vi "TOOLweb MESSWERTE.vi"(8 "error in (no error)":errorcluster caption="Fehler (Eingang, kein Fehler)", 9 "IP-Adresse (localhost)":string="127.0.0.1", 11 "Anzahl Gase":i32=18) -> (0 "Status":sgl[](array[numeric]), 1 "Diagnose":T2, 2 "gas#label":string[](array[string]), 5 "Zeitstempel":timestamp, 7 "Einstellungen":T1)   [LabVIEW 2020, in "FT-IR.lvlib" / "TOOLweb Interface.lvlib"]
doc: "Holt mit einer HTTP-POST-Anforderung gemäß TOOLweb-Protokoll die Gasmesswerte als Signalverläufe mit Gasnamen als Attribut \"NI_ChannelName\" und Zeitstempel vom MKS MultiGas 2030 Analyzer. Zwei Arrays mit den Gasnamen (Strings) und Gaskonzentrationsfehlern (DBL) werden zusätzlich bereitgestellt.\n\nAlle Daten werden zeitsparend in einem einzigen Poll Request zusammengefasst, damit nur einmal eine TCP/IP-Verbindung geöffnet werden muss.\n\nDer Ergebnis-Datentyp\"TOOLweb Signalverläufe\" ist als Typdefinitionen in der Bibliothek \"Datentypen\" enthalten\".\n\nFalls \"Anzahl Gase\" unverbunden bleibt, wird der Standardwert 18 verwendet.\n \nFalls der TOOLWeb-Server nicht auf demselben Rechner arbeitet, kann mit \"IP-Adresse\" eine beliebiger Host adressiert werden. Ein unverbundener Eingang spricht den lokalen Host an."
uses:
  TOOLweb Interface.lvlib
  TOOLweb Diagnose.ctl
  TOOLweb Einstellungen.ctl
  Stoerungen/Stoerungen Messgeraet/Aktionen Kommunikation Stoerung.ctl
  Get Spectra/Aktion FGV Background-Daten.ctl
  Aktion FGV Rezepte wechseln.ctl
  Span/Aktion FGV Span.ctl
  Aktionen EVID-Codes.ctl
  TOOLweb Interface Hilfs-VIs.lvlib
  Typdefinitionen.lvlib
  Stoerungen/Stoerungen.lvlib
  Get Spectra/Get Spectra.lvlib
  FT-IR.lvlib
  Span/Spanfaktor.lvlib
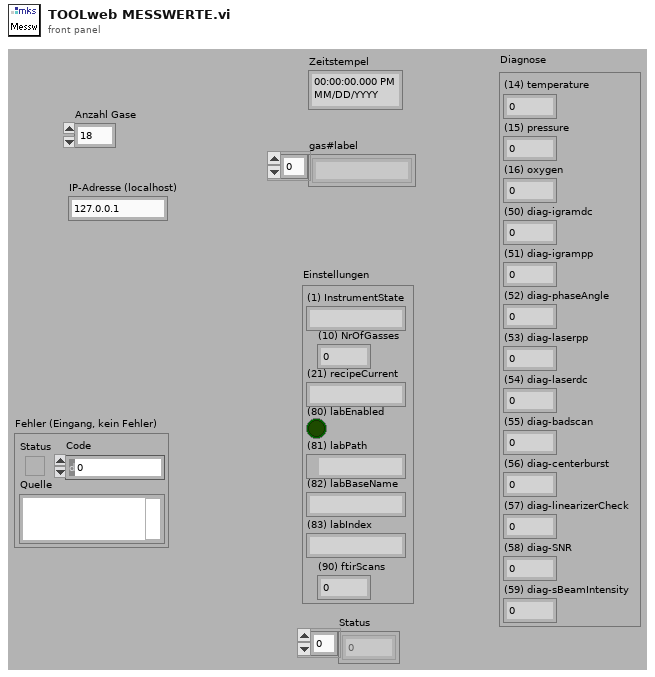
[diagram p1: front panel]
types:
  T1 = typedef "FT-IR.lvlib/TOOLweb Interface.lvlib/Typdefinitionen.lvlib/TOOLweb Einstellungen.ctl" = cluster{"(1) InstrumentState":string, "(10) NrOfGasses":i32, "(21) recipeCurrent":string, "(80) labEnabled":bool, "(81) labPath":path, "(82) labBaseName":string, "(83) labIndex":string, "(90) ftirScans":i32}
  T2 = typedef "FT-IR.lvlib/TOOLweb Interface.lvlib/Typdefinitionen.lvlib/TOOLweb Diagnose.ctl" = cluster{"(14) temperature":sgl, "(15) pressure":sgl, "(16) oxygen":sgl, "(50) diag-igramdc":sgl, "(51) diag-igrampp":sgl, "(52) diag-phaseAngle":sgl, "(53) diag-laserpp":sgl, "(54) diag-laserdc":sgl, "(55) diag-badscan":sgl, "(56) diag-centerburst":sgl, "(57) diag-linearizerCheck":sgl, "(58) diag-SNR":sgl, "(59) diag-sBeamIntensity":sgl}
  T3 = typedef "FT-IR.lvlib/Aktionen EVID-Codes.ctl" = enum16{"lesen", "setzen", "laden", "speichern", "1Hz/5Hz", "Smoothing", "Rolling Average"}
  T4 = typedef "FT-IR.lvlib/Spanfaktor.lvlib/Aktion FGV Span.ctl" = enum16{"lesen", "Span", "Seite aktiv", "Offset", "FGV aktualisiert", "Aktualisierung aufheben"}
  T5 = typedef "FT-IR.lvlib/Aktion FGV Rezepte wechseln.ctl" = enum16{"lesen", "Rezepte", "Rezeptindex", "Diesel", "Gasoline", "NCG", "laden", "speichern", "AK/Man"}
  T6 = typedef "FT-IR.lvlib/Get Spectra.lvlib/Aktion FGV Background-Daten.ctl" = enum16{"lesen", "schreiben", "Background aktiv", "Referenz", "laden", "speichern", "Plot sichtbar"}
  T7 = typedef "Stoerungen.lvlib/Aktionen Kommunikation Stoerung.ctl" = enum16{"lesen", "init", "FT-IR Komm", "FT-IR Betriebsart", "FT-IR Hintergrund", "cRIO Komm", "PNS Komm", "Dichtheitstest", "Life Bit", "FTIR Komm AK", "PMA Komm", "FID Komm", "PMA Cal", "FID Ch4 Cal", "FID THC Cal", "Cal Timeout", "VFS 1 Komm", "VFS 2 Komm", "VFS 3 Komm", "VFS 4 Komm", "TRE 08 Komm", "CG-Test vorzeitig", "CG-Test Span 1", "CG-Test Span 2", "CG-Test Span 3", "CG-Test Messgas", "CG-Test löschen", "Test", "Amium AK", "AK Recept konfig", "AK Name konfig", "AK EKFG konfig"}
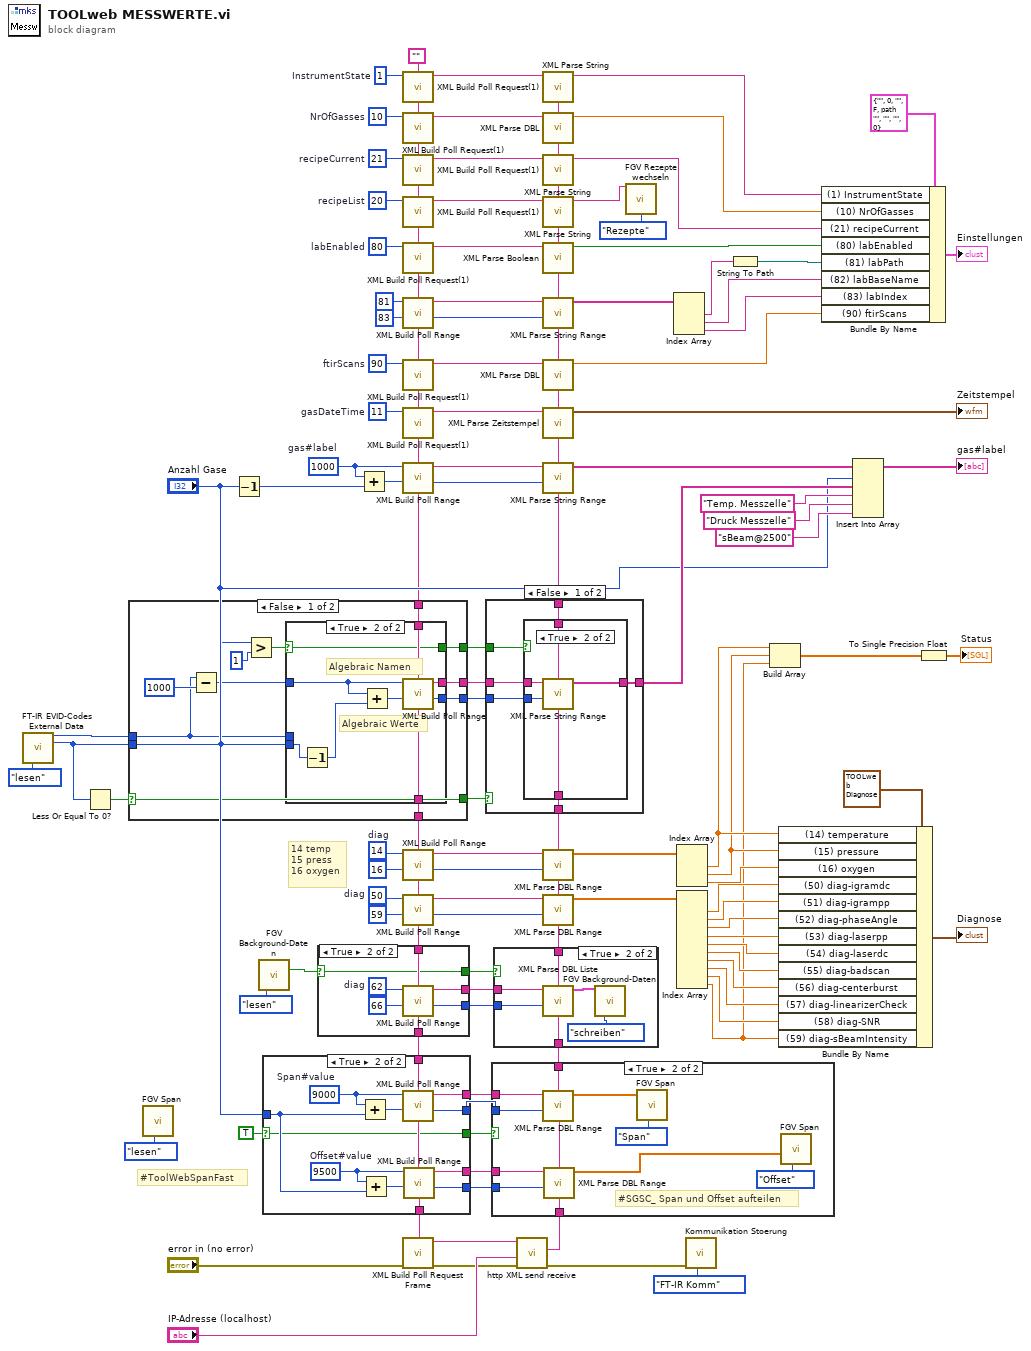
[diagram p0: block diagram]
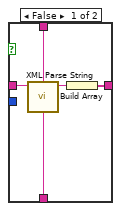
[diagram p2: hidden frame]
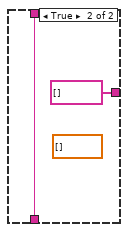
[diagram p3: hidden frame]
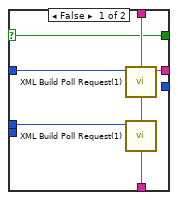
[diagram p4: hidden frame]
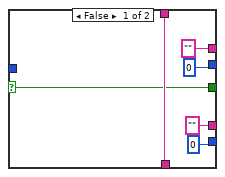
[diagram p7: hidden frame]
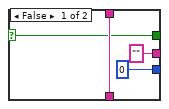
[diagram p9: hidden frame]
diagram:
  w29 = 20  # recipeList
  w54 = 14  # diag
  w81 = 90  # ftirScans
  w86 = 1  # InstrumentState
  w88 = 80  # labEnabled
  w89 = 21  # recipeCurrent
  w90 = 10  # NrOfGasses
  w103 = 50  # diag
  w126 = 1000  # gas#label
  w127 = 11  # gasDateTime
  # "#ToolWebSpanFast"
  # "14 temp\n15 press\n16 oxygen"
  n1 = call "FT-IR EVID-Codes External Data.vi"("Aktionen"=Aktionen_EVID-Codes."lesen") -> ("Startadresse"=w7:i32, "Anzahl"=w6:i32)  [unwired: 9 in, 4 out]
  n2 = Less Or Equal To 0?(x=w6) -> (x <= 0?=w5:bool)
  n3 = call "FGV Span.vi"("Aktion"=Aktion_FGV_Span."lesen") -> ()  [unwired: 7 in, 4 out]
  n4 = Decrement(x="Anzahl Gase") -> (x-1=w120:i32)
  n5 = call "FGV Background-Daten.vi"("Aktion"=Aktion_FGV_Background-Daten."lesen") -> ("Background aktiv"=w37:bool)  [unwired: 7 in, 7 out]
  n6 = Add(x=w126, y=w120) -> (x+y=w124:i32)
  n7 = call "XML Build Poll Request(1).vi"("XML-Message alt"="", "EVID-Nummer"=w86) -> ("Attribut Name"=w85:string, "XML-Message neu"=w78:string)  [unwired: 6 out]
  n8 = call "XML Build Poll Request(1).vi"("XML-Message alt"=w78, "EVID-Nummer"=w90) -> ("Attribut Name"=w91:string, "XML-Message neu"=w74:string)  [unwired: 6 out]
  n9 = call "XML Build Poll Request(1).vi"("XML-Message alt"=w74, "EVID-Nummer"=w89) -> ("Attribut Name"=w87:string, "XML-Message neu"=w28:string)  [unwired: 6 out]
  n10 = call "XML Build Poll Request(1).vi"("XML-Message alt"=w28, "EVID-Nummer"=w29) -> ("Attribut Name"=w30:string, "XML-Message neu"=w27:string)  [unwired: 6 out]
  n11 = call "XML Build Poll Request(1).vi"("XML-Message alt"=w27, "EVID-Nummer"=w88) -> ("Attribut Name"=w82:string, "XML-Message neu"=w61:string)  [unwired: 6 out]
  n12 = call "XML Build Poll Range.vi"("XML-Message alt"=w61, "von EVID-Nr"=81, "bis EVID-Nr"=83) -> ("Attribut Name (Range)"=w66:string, "Anzahl Elemente"=w67:i32, "XML-Message neu"=w59:string)  [unwired: 1 in, 3 out]
  n13 = call "XML Build Poll Request(1).vi"("XML-Message alt"=w59, "EVID-Nummer"=w81) -> ("Attribut Name"=w80:string, "XML-Message neu"=w70:string)  [unwired: 6 out]
  n14 = call "XML Build Poll Request(1).vi"("XML-Message alt"=w70, "EVID-Nummer"=w127) -> ("Attribut Name"=w125:string, "XML-Message neu"=w93:string)  [unwired: 6 out]
  n15 = call "XML Build Poll Range.vi"("XML-Message alt"=w93, "von EVID-Nr"=w126, "bis EVID-Nr"=w124) -> ("Attribut Name (Range)"=w123:string, "Anzahl Elemente"=w122:i32, "XML-Message neu"=w3:string)  [unwired: 1 in, 3 out]
  n16 = case shown="False" w5 {
    selector: w5 -> [w128 w157]
    tunnel: [w139 _] -> w10
    tunnel: [w138 _] -> w9
    tunnel: w3 -> [w137 w156]
    tunnel: [w136 w156] -> w45
    tunnel: [w133 _] -> w8
    tunnel: w7 -> [w131 _]
    tunnel: w6 -> [w129 _]
    tunnel: [w128 w157] -> w4
    frame False {
      n17 = Subtract(x=w131, y=1000) -> (x-y=w130:i32)
      n18 = Greater?(x=w129, y=1) -> (0:w135:bool)
      n19 = case shown="True" w135 {
        selector: w135 -> [w140 w151]
        tunnel: w131 -> [w146 _]
        tunnel: w129 -> [_ w149]
        tunnel: [w144 w155] -> w139
        tunnel: [_ w154] -> w138
        tunnel: w137 -> [w143 w152]
        tunnel: [w141 w147] -> w136
        tunnel: [w140 w151] -> w133
        tunnel: w130 -> [w145 w150]
        frame False {
          n20 = call "XML Build Poll Request(1).vi"("XML-Message alt"=w143, "EVID-Nummer"=w145) -> ("Attribut Name"=w144:string, "XML-Message neu"=w142:string)  [unwired: 6 out]
          n21 = call "XML Build Poll Request(1).vi"("XML-Message alt"=w142, "EVID-Nummer"=w146) -> ("XML-Message neu"=w141:string)  [unwired: 7 out]
        }
        frame True {
          # "Algebraic Werte"
          # "Algebraic Namen"
          n22 = Decrement(x=w149) -> (x-1=w148:i32)
          n23 = Add(x=w150, y=w148) -> (x+y=w153:i32)
          n24 = call "XML Build Poll Range.vi"("XML-Message alt"=w152, "von EVID-Nr"=w150, "bis EVID-Nr"=w153) -> ("Attribut Name (Range)"=w155:string, "Anzahl Elemente"=w154:i32, "XML-Message neu"=w147:string)  [unwired: 1 in, 3 out]
        }
      }
    }
    frame True {
    }
  }
  n25 = call "XML Build Poll Range.vi"("XML-Message alt"=w45, "von EVID-Nr"=w54, "bis EVID-Nr"=16) -> ("Attribut Name (Range)"=w52:string, "Anzahl Elemente"=w51:i32, "XML-Message neu"=w50:string)  [unwired: 1 in, 3 out]
  n26 = call "XML Build Poll Range.vi"("XML-Message alt"=w50, "von EVID-Nr"=w103, "bis EVID-Nr"=59) -> ("Attribut Name (Range)"=w105:string, "Anzahl Elemente"=w106:i32, "XML-Message neu"=w44:string)  [unwired: 1 in, 3 out]
  n27 = case shown="True" w37 {
    selector: w37 -> [w158 w162]
    tunnel: w44 -> [w161 w168]
    tunnel: [w161 w167] -> w22
    tunnel: ["" ("Attribut Name (Range)") w164] -> w39
    tunnel: [0 ("Anzahl Elemente") w163] -> w38
    tunnel: [w158 w162] -> w36
    frame False {
    }
    frame True {
      w166 = 62  # diag
      n28 = call "XML Build Poll Range.vi"("XML-Message alt"=w168, "von EVID-Nr"=w166, "bis EVID-Nr"=66) -> ("Attribut Name (Range)"=w164:string, "Anzahl Elemente"=w163:i32, "XML-Message neu"=w167:string)  [unwired: 1 in, 3 out]
    }
  }
  n29 = case shown="True" TRUE {
    selector: TRUE -> [w169 w175]
    tunnel: w22 -> [w174 w185]
    tunnel: ["" ("Attribut Name (Range)") w184] -> w20
    tunnel: [0 ("Anzahl Elemente") w183] -> w19
    tunnel: [0 ("Anzahl Elemente") w182] -> w18
    tunnel: ["" ("Attribut Name (Range)") w181] -> w17
    tunnel: [w174 w177] -> w15
    tunnel: "Anzahl Gase" -> [_ w176]
    tunnel: [w169 w175] -> w12
    frame False {
    }
    frame True {
      w180 = 9500  # Offset#value
      w186 = 9000  # Span#value
      n30 = Add(x=w186, y=w176) -> (x+y=w187:i32)
      n31 = Add(x=w180, y=w176) -> (x+y=w179:i32)
      n32 = call "XML Build Poll Range.vi"("XML-Message alt"=w185, "von EVID-Nr"=w186, "bis EVID-Nr"=w187) -> ("Attribut Name (Range)"=w184:string, "Anzahl Elemente"=w183:i32, "XML-Message neu"=w178:string)  [unwired: 1 in, 3 out]
      n33 = call "XML Build Poll Range.vi"("XML-Message alt"=w178, "von EVID-Nr"=w180, "bis EVID-Nr"=w179) -> ("Attribut Name (Range)"=w181:string, "Anzahl Elemente"=w182:i32, "XML-Message neu"=w177:string)  [unwired: 1 in, 3 out]
    }
  }
  n34 = call "XML Build Poll Request Frame.vi"("XML-Message"=w15, "error in (no error)"="error in (no error)") -> ("XML-Message fertig"=w40:string, "error out"=w41:errorcluster)  [unwired: 1 in, 5 out]
  n35 = call "http XML send receive.vi"("error in (no error)"=w41, "IP-Adresse (localhost)"="IP-Adresse (localhost)", "XML Request"=w40) -> ("error out"=w97:errorcluster, "Response Body (XML)"=w16:string)  [unwired: 3 out]
  n36 = case shown="True" w12 {
    tunnel: [w188 w199] -> w21
    tunnel: w20 -> [_ w198]
    tunnel: w19 -> [_ w197]
    tunnel: w18 -> [_ w196]
    tunnel: w17 -> [_ w195]
    tunnel: w16 -> [w188 w194]
    frame False {
    }
    frame True {
      # "#SGSC_ Span und Offset aufteilen"
      n37 = call "XML Parse DBL Range.vi"("Attribut Name"=w195, "XML Response"=w194, "Anzahl Elemente"=w196) -> ("Werte"=w190:dbl[], "XML Response gekürzt"=w193:string)  [unwired: 5 out]
      n38 = call "XML Parse DBL Range.vi"("Attribut Name"=w198, "XML Response"=w193, "Anzahl Elemente"=w197) -> ("Werte"=w192:dbl[], "XML Response gekürzt"=w199:string)  [unwired: 5 out]
      n39 = call "FGV Span.vi"("Aktion"=Aktion_FGV_Span."Span", "Span"=w192) -> ()  [unwired: 6 in, 4 out]
      n40 = call "FGV Span.vi"("Aktion"=Aktion_FGV_Span."Offset", "Offset"=w190) -> ()  [unwired: 6 in, 4 out]
    }
  }
  n41 = case shown="True" w36 {
    tunnel: [w200 w206] -> w43
    tunnel: w21 -> [w200 w205]
    tunnel: w39 -> [_ w204]
    tunnel: w38 -> [_ w203]
    frame False {
    }
    frame True {
      n42 = call "XML Parse DBL Liste.vi"("Attribut Name"=w204, "XML Response"=w205, "Anzahl Elemente"=w203) -> ("Background Daten"=w201:cluster{"Ramp Pattern":dbl[], dbl[]}[], "XML Response gekürzt"=w206:string)  [unwired: 5 in]
      n43 = call "FGV Background-Daten.vi"("Background Daten"=w201, "Aktion"=Aktion_FGV_Background-Daten."schreiben") -> ()  [unwired: 6 in, 8 out]
    }
  }
  n44 = call "XML Parse DBL Range.vi"("Attribut Name"=w105, "XML Response"=w43, "Anzahl Elemente"=w106) -> ("Werte"=w107:dbl[], "XML Response gekürzt"=w49:string)  [unwired: 5 out]
  n45 = call "XML Parse DBL Range.vi"("Attribut Name"=w52, "XML Response"=w49, "Anzahl Elemente"=w51) -> ("Werte"=w48:dbl[], "XML Response gekürzt"=w46:string)  [unwired: 5 out]
  n46 = case shown="False" w4 {
    tunnel: [w212 string[] [] ("Elemente (Strings)")] -> w47
    tunnel: [w211 w224] -> w2
    tunnel: w46 -> [w210 w224]
    tunnel: w10 -> [w209 _]
    tunnel: w9 -> [w208 _]
    tunnel: w8 -> [w207 _]
    frame False {
      n47 = case shown="True" w207 {
        tunnel: [w215 w222] -> w212
        tunnel: [w214 w221] -> w211
        tunnel: w210 -> [w213 w218]
        tunnel: w209 -> [w217 w220]
        tunnel: w208 -> [_ w219]
        frame False {
          n48 = call "XML Parse String.vi"("Attribut Name"=w217, "XML Response"=w213) -> ("Wert-String"=w216:string, "XML Response gekürzt"=w214:string)  [unwired: 6 out]
          n49 = Build Array(w216) -> (w215:string[])
        }
        frame True {
          n50 = call "XML Parse String Range.vi"("Attribut Name"=w220, "XML Response"=w218, "Anzahl Elemente"=w219) -> ("Elemente (Strings)"=w222:string[], "XML Response gekürzt"=w221:string)  [unwired: 5 out]
        }
      }
    }
    frame True {
      (unwired) dbl[] [] ("Werte")
    }
  }
  n51 = call "XML Parse String Range.vi"("Attribut Name"=w123, "XML Response"=w2, "Anzahl Elemente"=w122) -> ("Elemente (Strings)"=w101:string[], "XML Response gekürzt"=w92:string)  [unwired: 5 out]
  n52 = call "XML Parse Zeitstempel.vi"("Attribut Name"=w125, "XML Response"=w92) -> ("Zeitstempel"=→"Zeitstempel":timestamp, "XML Response gekürzt"=w69:string)  [unwired: 6 out]
  n53 = call "XML Parse DBL.vi"("Attribut Name"=w80, "XML Response"=w69) -> ("Wert (DBL)"=w68:dbl, "XML Response gekürzt"=w58:string)  [unwired: 6 out]
  n54 = call "XML Parse String Range.vi"("Attribut Name"=w66, "XML Response"=w58, "Anzahl Elemente"=w67) -> ("Elemente (Strings)"=w63:string[], "XML Response gekürzt"=w60:string)  [unwired: 5 out]
  n55 = call "XML Parse Boolean.vi"("Attribut Name"=w82, "XML Response"=w60) -> ("Wert (boolean)"=w77:bool, "XML Response gekürzt"=w25:string)  [unwired: 6 out]
  n56 = call "XML Parse String.vi"("Attribut Name"=w30, "XML Response"=w25) -> ("Wert-String"=w23:string, "XML Response gekürzt"=w26:string)  [unwired: 6 out]
  n57 = call "XML Parse String.vi"("Attribut Name"=w87, "XML Response"=w26) -> ("Wert-String"=w75:string, "XML Response gekürzt"=w73:string)  [unwired: 6 out]
  n58 = call "XML Parse DBL.vi"("Attribut Name"=w91, "XML Response"=w73) -> ("Wert (DBL)"=w83:dbl, "XML Response gekürzt"=w79:string)  [unwired: 6 out]
  n59 = call "XML Parse String.vi"("Attribut Name"=w85, "XML Response"=w79) -> ("Wert-String"=w84:string)  [unwired: 7 out]
  n60 = call "FGV Rezepte wechseln.vi"("Rezepte"=w23, "Aktion"=Aktion_FGV_Rezepte_wechseln."Rezepte") -> ()  [unwired: 7 in, 7 out]
  n61 = Index Array(array=w63) -> (element #1=w62:string, element #2=w56:string, element #3=w55:string)  [unwired: 3 in]
  n62 = Index Array(array=w48) -> (element #1=w34:dbl, element #2=w33:dbl, element #3=w102:dbl)  [unwired: 3 in]
  n63 = Index Array(array=w107) -> (element #1=w108:dbl, element #2=w109:dbl, element #3=w110:dbl, element #4=w111:dbl, element #5=w112:dbl, element #6=w113:dbl, element #7=w114:dbl, element #8=w115:dbl, element #9=w116:dbl, element #10=w31:dbl)  [unwired: 10 in]
  n64 = call "Kommunikation Stoerung.vi"("Aktionen"=Aktionen_Kommunikation_Stoerung."FT-IR Komm", "error in"=w97) -> ()  [unwired: 9 in, 1 out]
  n65 = String To Path(string=w62) -> (path=w57:path)
  n66 = Build Array(w34, w33, w31) -> (w32:dbl[])
  n67 = Bundle By Name(cluster=T2 {"(14) temperature"=0.0, "(15) pressure"=0.0, "(16) oxygen"=0.0, "(50) diag-igramdc"=0.0, "(51) diag-igrampp"=0.0, "(52) diag-phaseAngle"=0.0, "(53) diag-laserpp"=0.0, "(54) diag-laserdc"=0.0, "(55) diag-badscan"=0.0, "(56) diag-centerburst"=0.0, "(57) diag-linearizerCheck"=0.0, "(58) diag-SNR"=0.0, "(59) diag-sBeamIntensity"=0.0} ("Diagnose"), "(14) temperature"=w34, "(15) pressure"=w33, "(16) oxygen"=w102, "(50) diag-igramdc"=w108, "(51) diag-igrampp"=w109, "(52) diag-phaseAngle"=w110, "(53) diag-laserpp"=w111, "(54) diag-laserdc"=w112, "(55) diag-badscan"=w113, "(56) diag-centerburst"=w114, "(57) diag-linearizerCheck"=w115, "(58) diag-SNR"=w116, "(59) diag-sBeamIntensity"=w31) -> (→"Diagnose":T2)
  n68 = Bundle By Name(cluster=T1 {"(1) InstrumentState"="", "(10) NrOfGasses"=0, "(21) recipeCurrent"="", "(80) labEnabled"=FALSE, "(81) labPath"=path "", "(82) labBaseName"="", "(83) labIndex"="", "(90) ftirScans"=0} ("Info"), "(1) InstrumentState"=w84, "(10) NrOfGasses"=w83, "(21) recipeCurrent"=w75, "(80) labEnabled"=w77, "(81) labPath"=w57, "(82) labBaseName"=w56, "(83) labIndex"=w55, "(90) ftirScans"=w68) -> (→"Einstellungen":T1)
  n69 = Insert Into Array(array=w101, index="Anzahl Gase", new element #1=w47, new element #2="Temp. Messzelle" ("Neues Element/Teil-Array"), new element #3="Druck Messzelle" ("Neues Element/Teil-Array"), new element #4="sBeam@2500" ("Neues Element/Teil-Array")) -> (→"gas#label":string[])
  n70 = To Single Precision Float(number=w32) -> (single precision float=→"Status":sgl[])
